vi "Write Message.vi"(8 "error in (no error)":errorcluster, 10 "Message":string, 11 "CSV Test Log in":refnum<class "CSVOperationsLog.lvclass">) -> (0 "error out":errorcluster, 3 "CSV Test Log out":refnum<class "CSVOperationsLog.lvclass">)   [LabVIEW 2016, in "CSVOperationsLog.lvclass"]
uses:
  CSVOperationsLog.lvclass
  CSVOperationsLog.lvclass/CSVOperationsLog.ctl
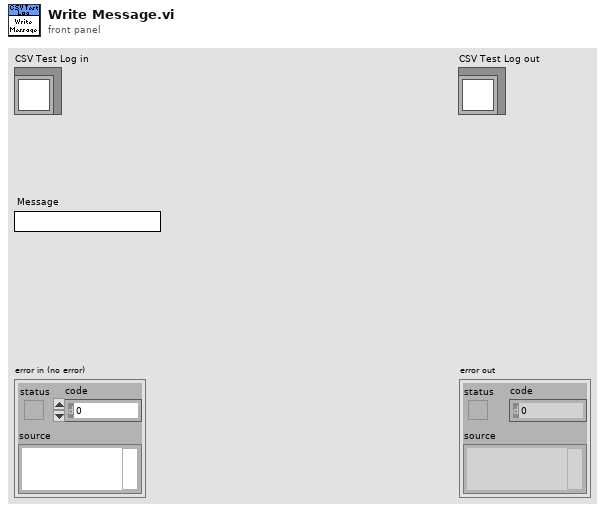
[diagram p1: front panel]
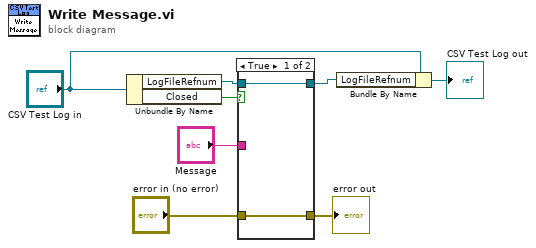
[diagram p0: block diagram]
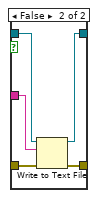
[diagram p2: hidden frame]
diagram:
  n1 = Unbundle By Name("CSV Test Log in") -> ("LogFileRefnum"=w8:refnum<file>, "Closed"=w1:bool)
  n2 = case shown="True" w1 {
    tunnel: w8 -> [w9 w15]
    tunnel: "Message" -> [_ w14]
    tunnel: "error in (no error)" -> [w10 w13]
    tunnel: [w10 w12] -> w5
    tunnel: [w9 w11] -> w2
    frame True {
    }
    frame False {
      n3 = Write to Text File(file (use dialog)=w15, text=w14, error in=w13) -> (refnum out=w11:refnum<file>, error out=w12:errorcluster)  [unwired: 1 in, 1 out]
    }
  }
  "error out" <- w5
  n4 = Bundle By Name(cluster="CSV Test Log in", "LogFileRefnum"=w2) -> (→"CSV Test Log out":refnum<class "CSVOperationsLog.lvclass">)
